vi "interface_configuration.vi"(8 "error in (no error)":errorcluster, 11 "config in":T1) -> (0 "error out":errorcluster, 3 "config out":T1)   [LabVIEW 2015, in "lv-builder.lvlib"]
uses:
  lv-builder.lvlib
  private/_controls/post_action_lvlib.ctl
  private/_controls/post_action_installer.ctl
  private/_controls/post_action_application.ctl
  private/_controls/post_action_zip.ctl
  _controls/configuration.ctl
  <vilib>/Utility/error.llb/Error Cluster From Error Code.vi
  <vilib>/ErrorRing/Error Ring.xnode
panel:
  in  "application_post_action":T2 caption="Application Post Action"
  in  "cancel":bool
  in  "save":bool
  in  "installer_post_file":path caption="Installer Post File"
  in  "zip_move_directory":path caption="Archive Directory"
  in  "zip_post_action":T3 caption="Archive Post Action"
  in  "installer_post_action":T4 caption="Installer Post Action"
  in  "update_version_vi":path caption="Update Version VI"
  in  "lvlibp_move_directory":path caption="lvlibp Directory"
  in  "lvlib_move_directory":path caption="lvlib Directory"
  in  "lvlib_post_action":T5 caption="LVLIB Post Action"
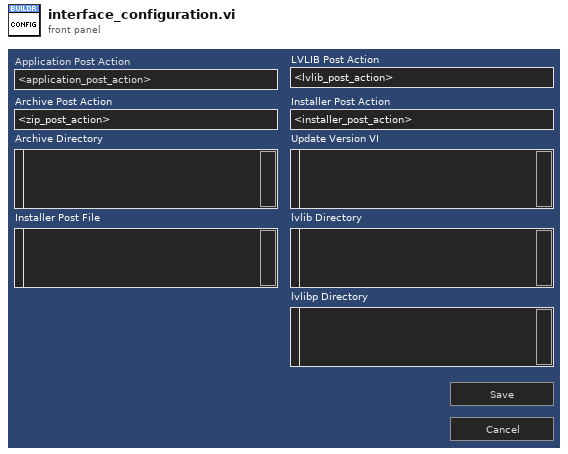
[diagram p1: front panel]
types:
  T1 = typedef "lv-builder.lvlib/configuration.ctl" = cluster{"lvlibp_directory":string, "zip_directory":string, "lvlib_directory":string, "update_version_vi":string, "installer_post_file":string, "lvlib_post_action":u16, "installer_post_action":u16, "application_post_action":u16, "zip_post_action":u16}
  T2 = typedef "lv-builder.lvlib/post_action_application.ctl" = enum16{"<application_post_action>", "nothing", "zip_application", "<null>"}
  T3 = typedef "lv-builder.lvlib/post_action_zip.ctl" = enum16{"<zip_post_action>", "nothing", "move", "extract", "<null>"}
  T4 = typedef "lv-builder.lvlib/post_action_installer.ctl" = enum16{"<installer_post_action>", "nothing", "create_installer", "zip_installer", "create_installer_file", "<null>"}
  T5 = typedef "lv-builder.lvlib/post_action_lvlib.ctl" = enum16{"<lvlib_post_action>", "nothing", "move", "install", "<null>"}
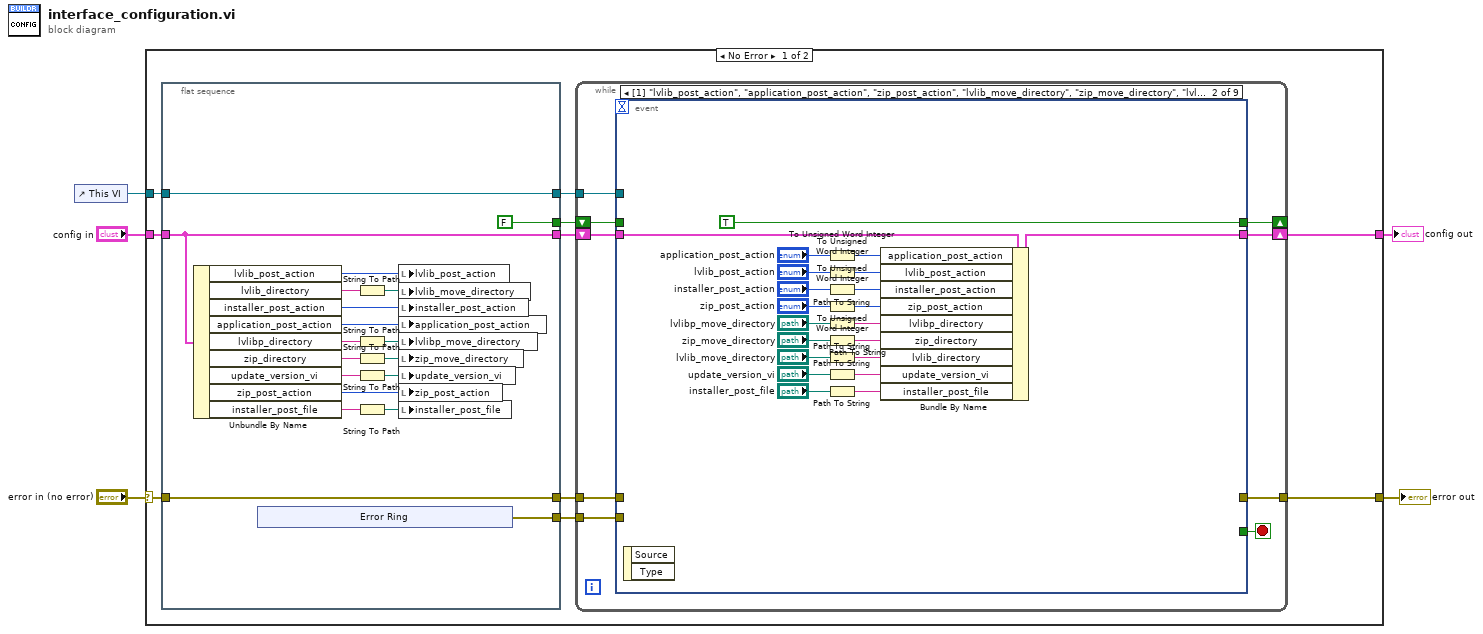
[diagram p0: block diagram]
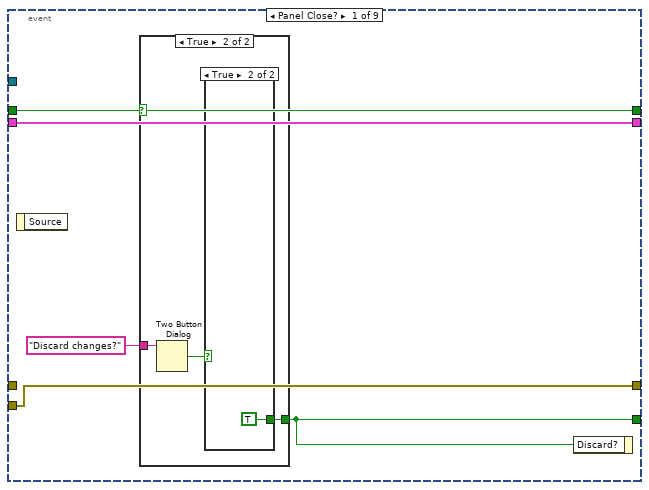
[diagram p2: hidden frame]
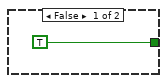
[diagram p3: hidden frame]
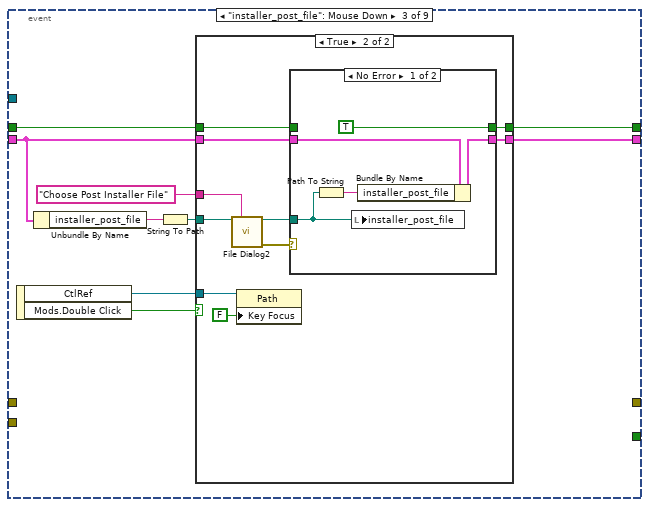
[diagram p5: hidden frame]
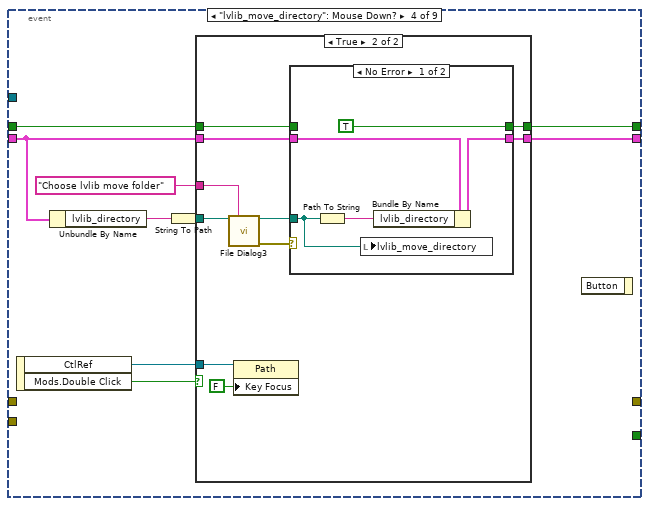
[diagram p8: hidden frame]
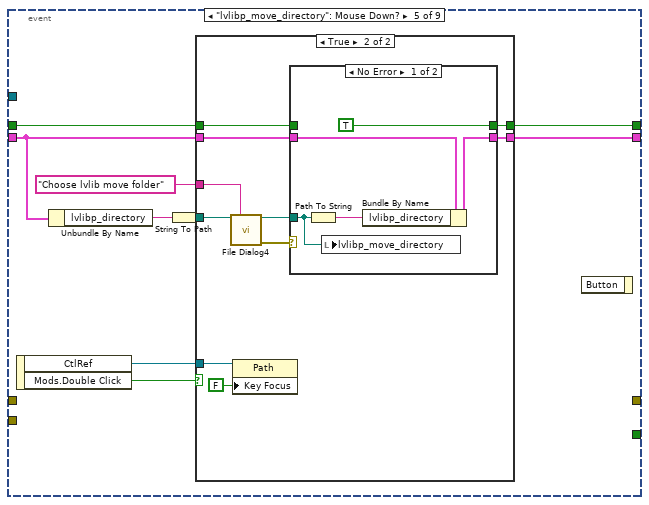
[diagram p11: hidden frame]
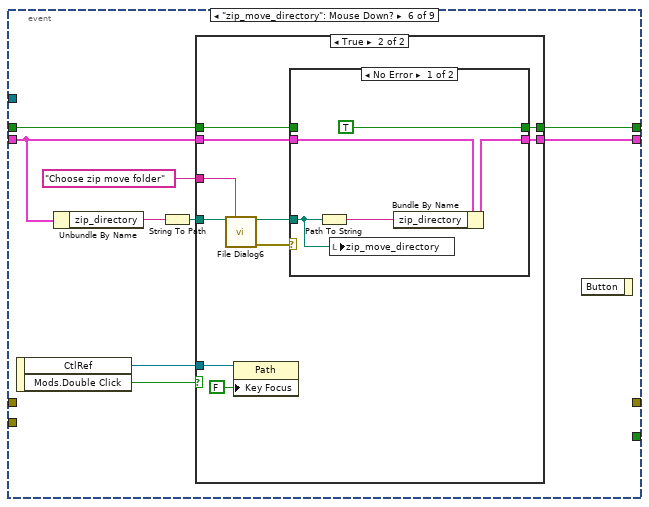
[diagram p14: hidden frame]
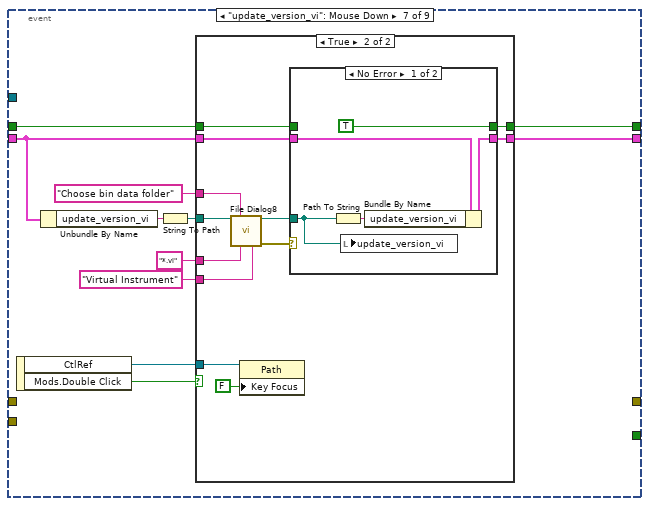
[diagram p17: hidden frame]
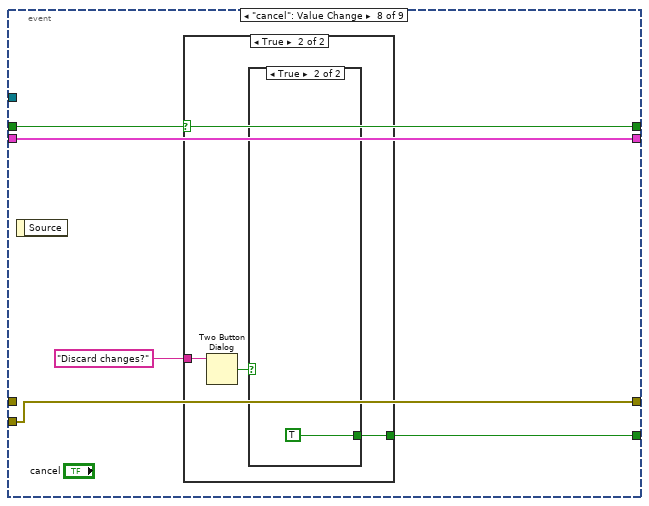
[diagram p20: hidden frame]
diagram:
  n1 = control-ref of="This VI"() -> (w3:refnum<vi>)
  n2 = case shown="No Error" "error in (no error)" {
    selector: "error in (no error)" -> [w15 w237]
    tunnel: [w9 w237] -> w4
    tunnel: w3 -> [w11 _]
    tunnel: [w8 _] -> w2
    tunnel: "config in" -> [w7 _]
    frame No Error {
      n3 = flat-sequence {
        tunnel: w15 -> [w17]
        tunnel: [w17] -> w14
        tunnel: [w18] -> w13
        tunnel: [w27] -> w12
        tunnel: w11 -> [w27]
        tunnel: [FALSE] -> w10
        tunnel: w7 -> [w18]
        tunnel: [w16] -> w6
        frame #0 {
          n4 = Unbundle By Name(w18) -> ("lvlib_post_action"=w28:u16, "lvlib_directory"=w33:string, "installer_post_action"=w29:u16, "application_post_action"=w30:u16, "lvlibp_directory"=w32:string, "zip_directory"=w31:string, "update_version_vi"=w26:string, "zip_post_action"=w25:u16, "installer_post_file"=w24:string)
          n5 = xnode "Error Ring"() -> ("error out"=w16:errorcluster)
          n6 = String To Path(string=w33) -> (path=w23:path)
          n7 = String To Path(string=w32) -> (path=w22:path)
          n8 = String To Path(string=w31) -> (path=w21:path)
          n9 = String To Path(string=w26) -> (path=w20:path)
          n10 = String To Path(string=w24) -> (path=w19:path)
          n11 = local write "lvlib_post_action"(w28) -> ()
          n12 = local write "lvlib_move_directory"(w23) -> ()
          n13 = local write "installer_post_action"(w29) -> ()
          n14 = local write "application_post_action"(w30) -> ()
          n15 = local write "lvlibp_move_directory"(w22) -> ()
          n16 = local write "zip_move_directory"(w21) -> ()
          n17 = local write "update_version_vi"(w20) -> ()
          n18 = local write "zip_post_action"(w25) -> ()
          n19 = local write "installer_post_file"(w19) -> ()
        }
      }
      n20 = while {
        tunnel: w14 -> [w40]
        shift-right: [w45] -> w8
        shift-left: w13 -> [w46]
        tunnel: w12 -> [w42]
        shift-right: [w43] -> _
        shift-left: w10 -> [w44]
        tunnel: [w41] -> w9
        tunnel: w6 -> [w39]
        stop <- w47 stop-if-true
        n21 = event shown="[1] \"lvlib_post_action\", \"application_post_action\", \"zip_post_action\", \"lvlib_move_directory\", \"zip_move_directory\", \"lvlibp_move_directory\", \"update_version_vi\", \"installer_post_file\", \"installer_post_action\": Value Change" {
          selector: _ -> [_ _ _ _ _ _ _ _ _]
          dyn-events: _ -> [_ _ _ _ _ _ _ _ _]
          timeout: _ -> [_ _ _ _ _ _ _ _ _]
          tunnel: [w50 _ _ _ _ _ _ w227 TRUE ("Discard?")] -> w47
          tunnel: w42 -> [_ _ _ _ _ _ _ _ _]
          tunnel: w46 -> [w52 w78 w83 w111 w139 w167 w197 w226 w235]
          tunnel: [w52 w76 w85 w113 w141 w169 w199 w226 w235] -> w45
          tunnel: w44 -> [w49 _ w87 w115 w143 w171 w201 w224 w236]
          tunnel: [w49 TRUE w86 w114 w142 w170 w200 w224 w236] -> w43
          tunnel: [w48 _ _ _ _ _ _ w223 w234] -> w41
          tunnel: w40 -> [_ _ _ _ _ _ _ _ w234]
          tunnel: w39 -> [w48 _ _ _ _ _ _ w223 _]
          event Panel Close? {
            n22 = event-data() -> ()  [unwired: 1 in, 1 out]
            n23 = case shown="True" w49 {
              tunnel: [TRUE ("Discard?") w56] -> w50
              tunnel: "Discard changes?" ("dialog_text") -> [_ w55]
              frame False {
              }
              frame True {
                n24 = Two Button Dialog(message=w55) -> (T button?=w54:bool)  [unwired: 2 in]
                n25 = case shown="True" w54 {
                  tunnel: [_ TRUE ("Discard?")] -> w56
                  frame False {
                  }
                  frame True {
                  }
                }
              }
            }
            n26 = event-data("Discard?"=w50) -> ()  [unwired: 1 in, 1 out]
          }
          event "lvlib_move_directory", "zip_move_directory", "lvlibp_move_directory", "update_version_vi", "installer_post_file": Value Change {
            n27 = event-data() -> ()  [unwired: 1 in, 2 out]
            n28 = To Unsigned Word Integer(number="application_post_action") -> (unsigned 16bit integer=w61:u16)
            n29 = To Unsigned Word Integer(number="lvlib_post_action") -> (unsigned 16bit integer=w60:u16)
            n30 = To Unsigned Word Integer(number="installer_post_action") -> (unsigned 16bit integer=w59:u16)
            n31 = To Unsigned Word Integer(number="zip_post_action") -> (unsigned 16bit integer=w58:u16)
            n32 = Path To String(path="lvlibp_move_directory") -> (string=w66:string)
            n33 = Path To String(path="zip_move_directory") -> (string=w65:string)
            n34 = Path To String(path="lvlib_move_directory") -> (string=w64:string)
            n35 = Path To String(path="update_version_vi") -> (string=w63:string)
            n36 = Path To String(path="installer_post_file") -> (string=w62:string)
            n37 = Bundle By Name(cluster=w78, "application_post_action"=w61, "lvlib_post_action"=w60, "installer_post_action"=w59, "zip_post_action"=w58, "lvlibp_directory"=w66, "zip_directory"=w65, "lvlib_directory"=w64, "update_version_vi"=w63, "installer_post_file"=w62) -> (w76:T1)
          }
          event "installer_post_file": Mouse Down {
            n38 = event-data() -> ("CtlRef"=w79:refnum<vi>, "Mods.Double Click"=w84:bool)  [unwired: 1 in]
            n39 = Unbundle By Name(w83) -> ("installer_post_file"=w82:string)
            n40 = String To Path(string=w82) -> (path=w80:path)
            n41 = case shown="True" w84 {
              tunnel: w87 -> [w89 w99]
              tunnel: w83 -> [w88 w98]
              tunnel: [w89 w97] -> w86
              tunnel: [w88 w96] -> w85
              tunnel: w80 -> [_ w95]
              tunnel: "Choose Post Installer File" ("description") -> [_ w94]
              tunnel: w79 -> [_ w91]
              frame False {
              }
              frame True {
                n42 = call "File Dialog2"("start path"=w95, "prompt"=w94) -> ("selected path"=w93:path, "error out"=w92:errorcluster)  [unwired: 10 in, 2 out]
                n43 = property class="Path"(reference=w91, "Key Focus"=FALSE) -> ()  [unwired: 1 in, 2 out]
                n44 = case shown="No Error" w92 {
                  tunnel: w99 -> [_ w106]
                  tunnel: w98 -> [w103 w105]
                  tunnel: [TRUE w106] -> w97
                  tunnel: [w102 w105] -> w96
                  tunnel: w93 -> [w100 _]
                  frame No Error {
                    n45 = Path To String(path=w100) -> (string=w101:string)
                    n46 = local write "installer_post_file"(w100) -> ()
                    n47 = Bundle By Name(cluster=w103, "installer_post_file"=w101) -> (w102:T1)
                  }
                  frame Error {
                  }
                }
              }
            }
          }
          event "lvlib_move_directory": Mouse Down? {
            n48 = event-data() -> ("CtlRef"=w107:refnum<vi>, "Mods.Double Click"=w112:bool)  [unwired: 1 in]
            n49 = Unbundle By Name(w111) -> ("lvlib_directory"=w110:string)
            n50 = String To Path(string=w110) -> (path=w108:path)
            n51 = case shown="True" w112 {
              tunnel: w115 -> [w117 w127]
              tunnel: w111 -> [w116 w126]
              tunnel: [w117 w125] -> w114
              tunnel: [w116 w124] -> w113
              tunnel: w108 -> [_ w122]
              tunnel: "Choose lvlib move folder" ("description") -> [_ w123]
              tunnel: w107 -> [_ w118]
              frame False {
              }
              frame True {
                n52 = call "File Dialog3"("start path"=w122, "prompt"=w123) -> ("selected path"=w121:path, "error out"=w120:errorcluster)  [unwired: 10 in, 2 out]
                n53 = property class="Path"(reference=w118, "Key Focus"=FALSE) -> ()  [unwired: 1 in, 2 out]
                n54 = case shown="No Error" w120 {
                  tunnel: w127 -> [_ w134]
                  tunnel: w126 -> [w131 w133]
                  tunnel: [TRUE w134] -> w125
                  tunnel: [w130 w133] -> w124
                  tunnel: w121 -> [w129 _]
                  frame No Error {
                    n55 = Path To String(path=w129) -> (string=w128:string)
                    n56 = local write "lvlib_move_directory"(w129) -> ()
                    n57 = Bundle By Name(cluster=w131, "lvlib_directory"=w128) -> (w130:T1)
                  }
                  frame Error {
                  }
                }
              }
            }
            n58 = event-data() -> ()  [unwired: 2 in, 1 out]
          }
          event "lvlibp_move_directory": Mouse Down? {
            n59 = event-data() -> ("CtlRef"=w135:refnum<vi>, "Mods.Double Click"=w140:bool)  [unwired: 1 in]
            n60 = Unbundle By Name(w139) -> ("lvlibp_directory"=w138:string)
            n61 = String To Path(string=w138) -> (path=w136:path)
            n62 = case shown="True" w140 {
              tunnel: w143 -> [w145 w155]
              tunnel: w139 -> [w144 w154]
              tunnel: [w145 w153] -> w142
              tunnel: [w144 w152] -> w141
              tunnel: w136 -> [_ w150]
              tunnel: "Choose lvlib move folder" ("description") -> [_ w148]
              tunnel: w135 -> [_ w146]
              frame False {
              }
              frame True {
                n63 = call "File Dialog4"("start path"=w150, "prompt"=w148) -> ("selected path"=w149:path, "error out"=w151:errorcluster)  [unwired: 10 in, 2 out]
                n64 = property class="Path"(reference=w146, "Key Focus"=FALSE) -> ()  [unwired: 1 in, 2 out]
                n65 = case shown="No Error" w151 {
                  tunnel: w155 -> [_ w162]
                  tunnel: w154 -> [w159 w161]
                  tunnel: [TRUE w162] -> w153
                  tunnel: [w158 w161] -> w152
                  tunnel: w149 -> [w157 _]
                  frame No Error {
                    n66 = Path To String(path=w157) -> (string=w156:string)
                    n67 = local write "lvlibp_move_directory"(w157) -> ()
                    n68 = Bundle By Name(cluster=w159, "lvlibp_directory"=w156) -> (w158:T1)
                  }
                  frame Error {
                  }
                }
              }
            }
            n69 = event-data() -> ()  [unwired: 2 in, 1 out]
          }
          event "zip_move_directory": Mouse Down? {
            n70 = event-data() -> ("CtlRef"=w163:refnum<vi>, "Mods.Double Click"=w168:bool)  [unwired: 1 in]
            n71 = Unbundle By Name(w167) -> ("zip_directory"=w166:string)
            n72 = String To Path(string=w166) -> (path=w164:path)
            n73 = case shown="True" w168 {
              tunnel: w171 -> [w173 w183]
              tunnel: w167 -> [w172 w182]
              tunnel: [w173 w181] -> w170
              tunnel: [w172 w180] -> w169
              tunnel: w164 -> [_ w178]
              tunnel: "Choose zip move folder" ("description") -> [_ w177]
              tunnel: w163 -> [_ w174]
              frame False {
              }
              frame True {
                n74 = call "File Dialog6"("start path"=w178, "prompt"=w177) -> ("selected path"=w179:path, "error out"=w176:errorcluster)  [unwired: 10 in, 2 out]
                n75 = property class="Path"(reference=w174, "Key Focus"=FALSE) -> ()  [unwired: 1 in, 2 out]
                n76 = case shown="No Error" w176 {
                  tunnel: w183 -> [_ w190]
                  tunnel: w182 -> [w187 w189]
                  tunnel: [TRUE w190] -> w181
                  tunnel: [w186 w189] -> w180
                  tunnel: w179 -> [w185 _]
                  frame No Error {
                    n77 = Path To String(path=w185) -> (string=w184:string)
                    n78 = local write "zip_move_directory"(w185) -> ()
                    n79 = Bundle By Name(cluster=w187, "zip_directory"=w184) -> (w186:T1)
                  }
                  frame Error {
                  }
                }
              }
            }
            n80 = event-data() -> ()  [unwired: 2 in, 1 out]
          }
          event "update_version_vi": Mouse Down {
            n81 = event-data() -> ("CtlRef"=w191:refnum<vi>, "Mods.Double Click"=w198:bool)  [unwired: 1 in]
            n82 = Unbundle By Name(w197) -> ("update_version_vi"=w196:string)
            n83 = String To Path(string=w196) -> (path=w194:path)
            n84 = case shown="True" w198 {
              tunnel: w201 -> [w203 w215]
              tunnel: w197 -> [w202 w214]
              tunnel: [w203 w213] -> w200
              tunnel: [w202 w212] -> w199
              tunnel: w194 -> [_ w211]
              tunnel: "Choose bin data folder" ("description") -> [_ w208]
              tunnel: "*.vi" ("filter") -> [_ w207]
              tunnel: "Virtual Instrument" ("filter") -> [_ w206]
              tunnel: w191 -> [_ w204]
              frame False {
              }
              frame True {
                n85 = call "File Dialog8"("start path"=w211, "prompt"=w208, "pattern (all files)"=w207, "pattern label"=w206) -> ("selected path"=w210:path, "error out"=w209:errorcluster)  [unwired: 8 in, 2 out]
                n86 = property class="Path"(reference=w204, "Key Focus"=FALSE) -> ()  [unwired: 1 in, 2 out]
                n87 = case shown="No Error" w209 {
                  tunnel: w215 -> [_ w222]
                  tunnel: w214 -> [w219 w221]
                  tunnel: [TRUE w222] -> w213
                  tunnel: [w218 w221] -> w212
                  tunnel: w210 -> [w217 _]
                  frame No Error {
                    n88 = Path To String(path=w217) -> (string=w216:string)
                    n89 = local write "update_version_vi"(w217) -> ()
                    n90 = Bundle By Name(cluster=w219, "update_version_vi"=w216) -> (w218:T1)
                  }
                  frame Error {
                  }
                }
              }
            }
          }
          event "cancel": Value Change {
            n91 = event-data() -> ()  [unwired: 1 in, 1 out]
            n92 = case shown="True" w224 {
              tunnel: [TRUE ("Discard?") w231] -> w227
              tunnel: "Discard changes?" ("dialog_text") -> [_ w229]
              frame False {
              }
              frame True {
                n93 = Two Button Dialog(message=w229) -> (T button?=w230:bool)  [unwired: 2 in]
                n94 = case shown="True" w230 {
                  tunnel: [_ TRUE ("Discard?")] -> w231
                  frame False {
                  }
                  frame True {
                  }
                }
              }
            }
          }
          event "save": Value Change {
            n95 = event-data() -> ()  [unwired: 1 in, 1 out]
          }
        }
      }
    }
    frame Error {
    }
  }
  "error out" <- w4
  "config out" <- w2
